vi "SL2_AD_DLL_Phoibos_SetVoltage.vi"(5 "commit":bool, 6 "pHandle":u32, 7 "error in":errorcluster, 8 "value":dbl, 9 "voltageName":string, 10 "dll path in":path) -> (0 "error out":errorcluster, 3 "dll path out":path)   [LabVIEW 2020]
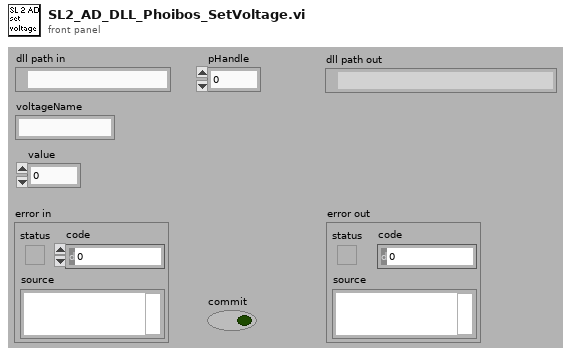
[diagram p1: front panel]
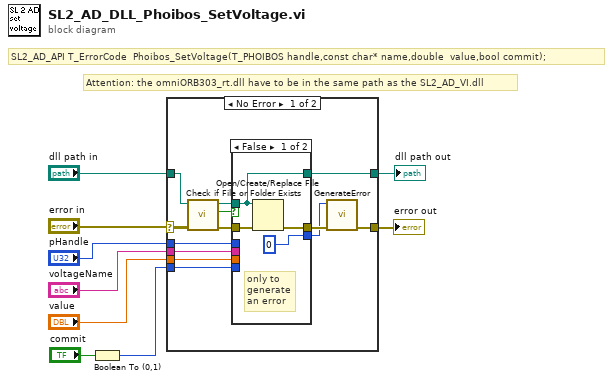
[diagram p0: block diagram]
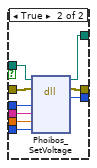
[diagram p2: hidden frame]
diagram:
  # "SL2_AD_API T_ErrorCode  Phoibos_SetVoltage(T_PHOIBOS handle,const char* name,double  value,bool commit);"
  # "Attention: the omniORB303_rt.dll have to be in the same path as the SL2_AD_VI.dll"
  n1 = Boolean To (0,1)(Boolean="commit") -> (0, 1=w1:i16)
  n2 = case shown="No Error" "error in" {
    selector: "error in" -> [w21 w36]
    tunnel: [w14 w36] -> w9
    tunnel: [w22 w37] -> w8
    tunnel: "dll path in" -> [w20 w37]
    tunnel: w1 -> [w19 _]
    tunnel: "pHandle" -> [w18 _]
    tunnel: "voltageName" -> [w17 _]
    tunnel: "value" -> [w16 _]
    frame No Error {
      n3 = call <vilib>:"Check if File or Folder Exists.vi"("error in (no error)"=w21, "path"=w20) -> ("error out"=w10:errorcluster, "file or folder exists?"=w12:bool, "dup path"=w11:path)  [unwired: 7 in]
      n4 = case shown="False" w12 {
        tunnel: [w25 w32] -> w15
        tunnel: [u32 0 ("error_code") w31] -> w13
        tunnel: [w24 w33] -> w22
        tunnel: w11 -> [w24 w35]
        tunnel: w10 -> [w26 w34]
        tunnel: w19 -> [_ w30]
        tunnel: w18 -> [_ w27]
        tunnel: w16 -> [_ w29]
        tunnel: w17 -> [_ w28]
        frame False {
          # "only to generate an error"
          n5 = Open/Create/Replace File(file path (use dialog)=w24, error in=w26) -> (error out=w25:errorcluster)  [unwired: 4 in, 2 out]
        }
        frame True {
          n6 = dll-call lib="C:/Programme/SPECS/SpecsLab2/programming/LabView7.1/SL2_AD_VI.dll" fn="Phoibos_SetVoltage" ("SetVoltage")(path in=w35, error in=w34, "pHandle"=w27, "voltageName"=w28, "value"=w29, "commit"=w30) -> (path out=w33:path, error out=w32:errorcluster, "error_code"=w31:u32)  [unwired: 5 in]
        }
      }
      n7 = call "GenerateError.vi"("error in"=w15, "error_code"=w13) -> ("error out"=w14:errorcluster)  [unwired: 9 in]
    }
    frame Error {
    }
  }
  "error out" <- w9
  "dll path out" <- w8
